vi "Down Hole CAL_PRESSURE_TRANSDUCER 2016.vi"(0 "Distance from APS Tip to transducer (ft)":dbl=5.2 format="%.2f", 2 "Sensor Cluster":T1, 3 "Descriptions":string[](array[string]), 5 "error in (no error)":errorcluster, 8 "Array in":refnum<k24>[](array[refnum])) -> (7 "DHT Zero (V)":dbl format="%.2f", 9 "DHT 10psi  (V)":dbl format="%.2f", 10 "Array out":refnum<k24>[](array[refnum]), 11 "DHT 50psi  (V)":dbl format="%.2f", 12 "Distance from APS Tip to transducer out":dbl=5.2 format="%.2f", 14 "Pressure\nSlope (psi/V)":dbl format="%.2f", 15 "Pressure\nOffset (psi)":dbl format="%.2f", 16 "Sensor Cluster 2":T1, 19 "error out":errorcluster)   [LabVIEW 2016]
uses:
  controls/MCC DAQ Readings.ctl
  C:/Cascade-lv16-64/builds/Waterloo Main Program/cascade/data/ULx_LV.dll
  builds/Waterloo Main Program/cascade/data/ULx_LV.dll
  Kpro Globals.vi
panel:
  in  "Exit":bool
  in  "50psi Pressure (psi)":dbl format="%.2f"
  in  "10psi Up Pressure (psi)":dbl format="%.2f"
  out "50psi indicator":bool
  in  "50psi button":bool
  out "Loop Counter":i32
  out "10psi\nindicator":bool
  out "zero indicator":bool
  in  "10psi button":bool
  in  "zero button":bool
  # "DOWNHOLE PRESSURE TRANSDUCER CALIBRATION"
  # "1. Connect the transducer to the KPRO line with the 3 way valve connected to the effluent of the transducer.  \n2.  Enter the distance from the APS tip to the transducer.\n3.  With the flow off, select the \"Record Zero Pressure\" button."
  # "3. Set the regulator pressure to a value close to 10psi, turn on the flow, close the 3-way valve and wait for the pressure to stabilize.  When it is stable, enter the \"10psi Pressure\" control, and select the \"Record ~10psi Voltage\" button."
  # "4. Set the regulator pressure to a value close to 50psi, turn on the flow, close the 3-way valve and wait for the pressure to stabilize.  When it is stable, enter the \"50psi Pressure\" control, and select the \"Record ~50psi Voltage\" button."
  # "5.  Slope and offset will be calculated, automatically.\nRecord the values for zero, slope and offset to the logbook and to the paper field log, then select the \"Record Values and Exit\" button."
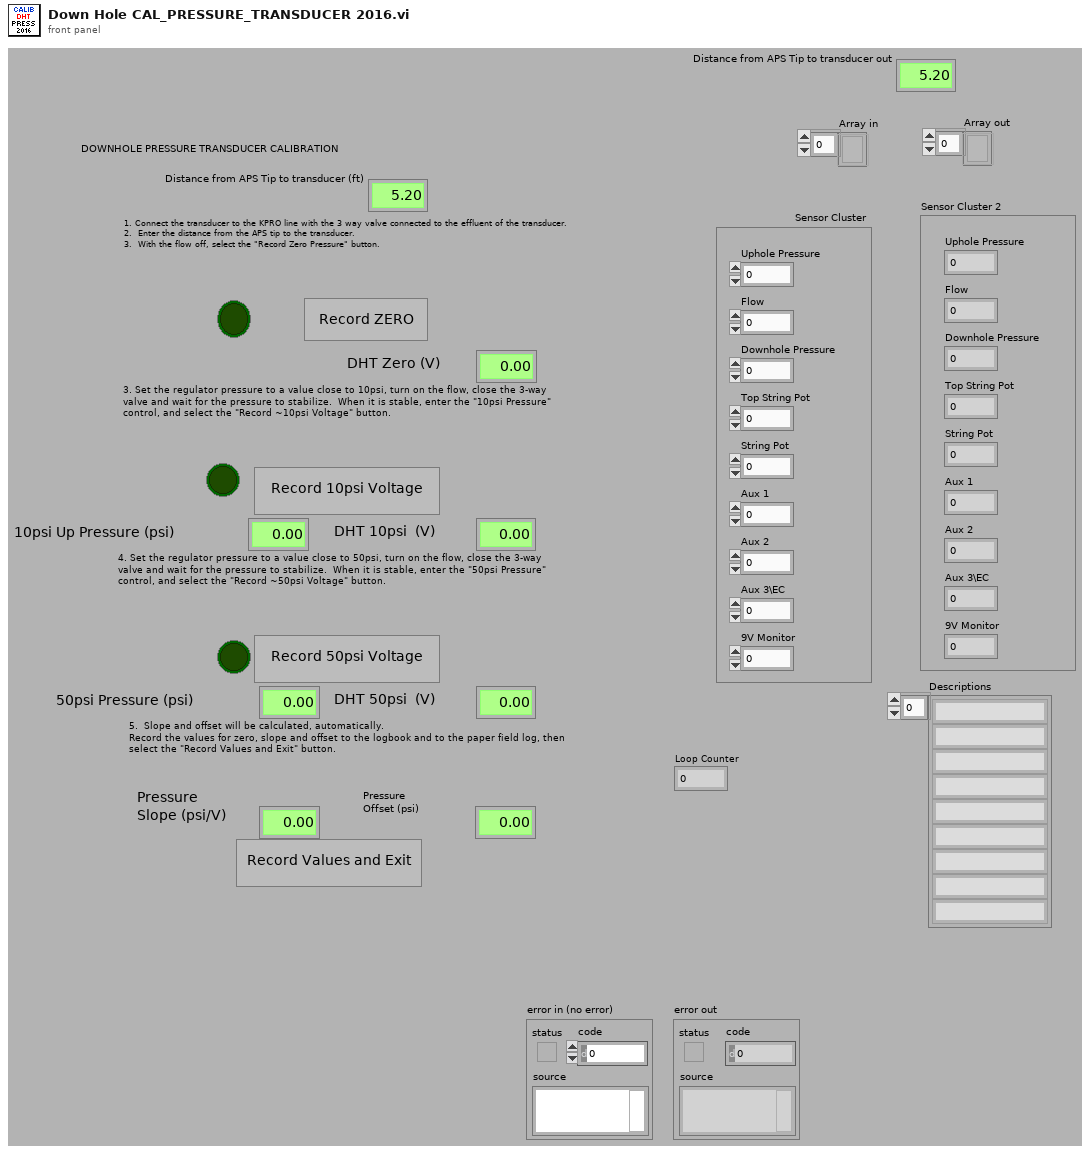
[diagram p1: front panel]
types:
  T1 = typedef "MCC DAQ Readings.ctl" = cluster{"Uphole Pressure":dbl, "Flow":dbl, "Downhole Pressure":dbl, "Top String Pot":dbl, "String Pot":dbl, "Aux 1":dbl, "Aux 2":dbl, "Aux 3\\EC":dbl, "9V Monitor":dbl}
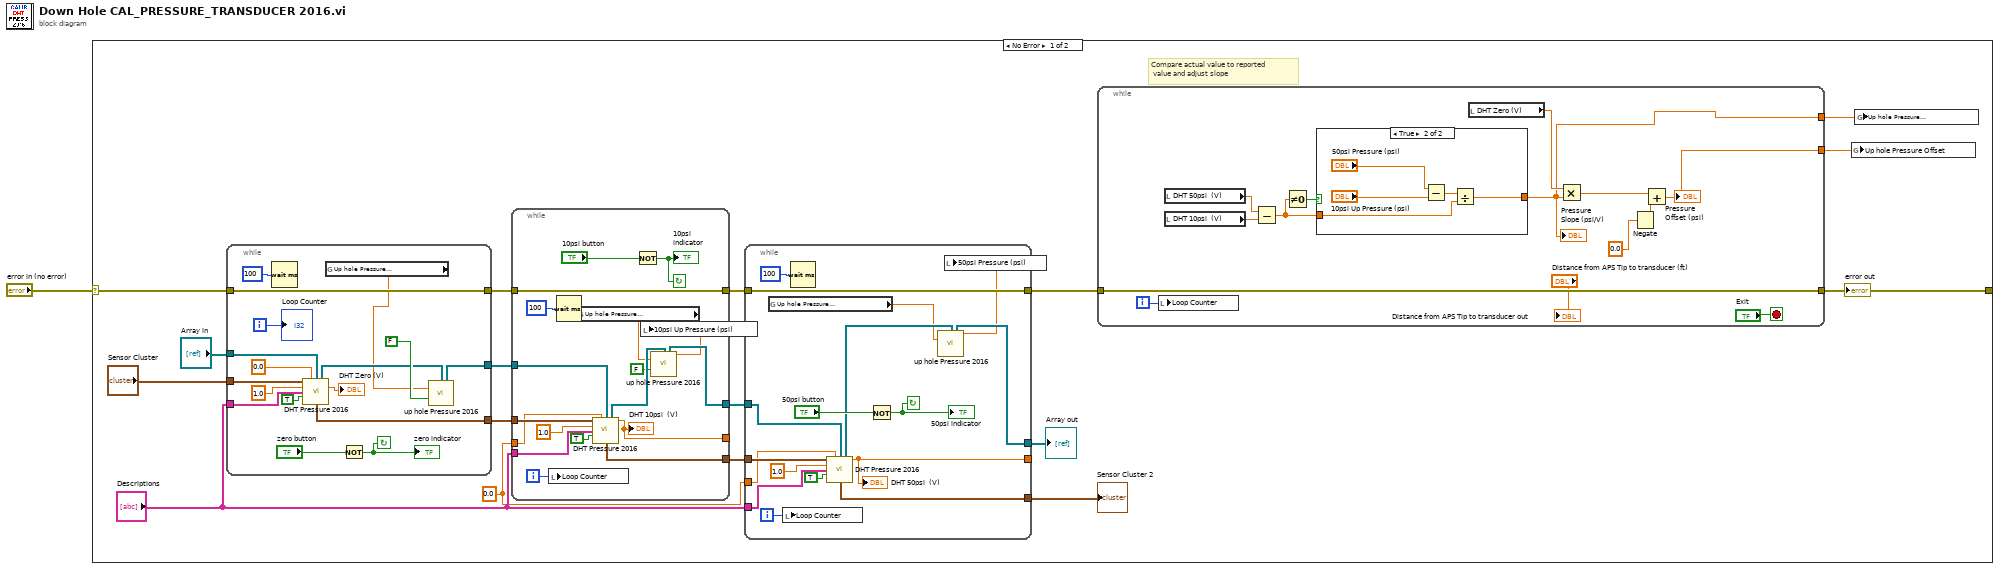
[diagram p0: block diagram]
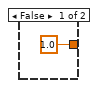
[diagram p2: hidden frame]
diagram:
  n1 = case shown="No Error" "error in (no error)" {
    selector: "error in (no error)" -> [w19 w92]
    tunnel: [w6 w92] -> w2
    frame No Error {
      w5 = 0.0
      # "Compare actual value to reported\n value and adjust slope"
      n2 = while {
        tunnel: [w72] -> w18
        tunnel: w19 -> [w72]
        tunnel: "Sensor Cluster" -> [w69]
        tunnel: "Array in" -> [w68]
        tunnel: [w58] -> w16
        tunnel: "Descriptions" -> [w67]
        tunnel: [w66] -> w14
        i -> [w62]
        stop <- w70 continue-if-true
        n3 = Wait (ms)(milliseconds to wait=u32 100) -> ()  [unwired: 1 out]
        n4 = call "DHT Pressure 2016.vi"("Sensor Cluster"=w69, "DHT Pressure Offset"=0.0, "Array in"=w68, "DHT Pressure \nSlope"=1.0 ("DHT Pressure \nSlope"), "Descriptions"=w67, "Zero Pressure\n(F = leave as is)"=TRUE ("Zero Pressure\n(F = leave as is)")) -> ("Array out"=w59:refnum<k24>[], "DHT Pressure (V)"=→"DHT Zero (V)":dbl, "Sensor Cluster 2"=w66:T1)  [unwired: 6 in, 1 out]
        n5 = global read "Kpro Globals.vi" "Up hole Pressure \nSlope"() -> (w57:dbl)
        n6 = Not(x="zero button") -> (.not. x?=w70:bool)
        "zero indicator" <- w70
        n7 = call "up hole Pressure 2016.vi"("Array in"=w59, "Pressure \nSlope"=w57, "Zero Pressure\n(F = leave as is)"=FALSE ("Zero Pressure\n(F = leave as is)")) -> ("Array out"=w58:refnum<k24>[])  [unwired: 9 in, 3 out]
        "Loop Counter" <- w62
      }
      n8 = while {
        tunnel: [w82] -> _
        tunnel: w18 -> [w90]
        tunnel: [w90] -> w13
        tunnel: w16 -> [w87]
        tunnel: [w77] -> w9
        tunnel: "Descriptions" -> [w86]
        tunnel: w14 -> [w85]
        tunnel: [w84] -> w12
        tunnel: w5 -> [w79]
        i -> [w80]
        stop <- w88 continue-if-true
        n9 = local write "Loop Counter"(w80) -> ()
        n10 = Wait (ms)(milliseconds to wait=u32 100) -> ()  [unwired: 1 out]
        n11 = global read "Kpro Globals.vi" "Up hole Pressure \nSlope"() -> (w76:dbl)
        n12 = call "DHT Pressure 2016.vi"("Sensor Cluster"=w85, "DHT Pressure Offset"=w79, "Array in"=w87, "DHT Pressure \nSlope"=1.0 ("DHT Pressure \nSlope"), "Descriptions"=w86, "Zero Pressure\n(F = leave as is)"=TRUE ("Zero Pressure\n(F = leave as is)")) -> ("Array out"=w78:refnum<k24>[], "DHT Pressure (ft/H20)"=w82:dbl, "Sensor Cluster 2"=w84:T1)  [unwired: 6 in, 1 out]
        "DHT 10psi  (V)" <- w82
        n13 = Not(x="10psi button") -> (.not. x?=w88:bool)
        "10psi\nindicator" <- w88
        n14 = call "up hole Pressure 2016.vi"("Array in"=w78, "Pressure \nSlope"=w76, "Zero Pressure\n(F = leave as is)"=FALSE ("Zero Pressure\n(F = leave as is)")) -> ("Array out"=w77:refnum<k24>[], "Uphole Pressure"=w74:dbl)  [unwired: 9 in, 2 out]
        n15 = local write "10psi Up Pressure (psi)"(w74) -> ()
      }
      n16 = while {
        tunnel: [w45] -> _
        tunnel: w13 -> [w56]
        tunnel: [w56] -> w7
        tunnel: w9 -> [w54]
        tunnel: [w43] -> w8
        tunnel: "Descriptions" -> [w53]
        tunnel: w12 -> [w52]
        tunnel: [w51] -> w10
        tunnel: w5 -> [w44]
        i -> [w46]
        stop <- w48 continue-if-true
        n17 = global read "Kpro Globals.vi" "Up hole Pressure \nSlope"() -> (w41:dbl)
        n18 = local write "Loop Counter"(w46) -> ()
        n19 = Wait (ms)(milliseconds to wait=u32 100) -> ()  [unwired: 1 out]
        n20 = call "DHT Pressure 2016.vi"("Sensor Cluster"=w52, "DHT Pressure Offset"=w44, "Array in"=w54, "DHT Pressure \nSlope"=1.0 ("DHT Pressure \nSlope"), "Descriptions"=w53, "Zero Pressure\n(F = leave as is)"=TRUE ("Zero Pressure\n(F = leave as is)")) -> ("Array out"=w42:refnum<k24>[], "DHT Pressure (ft/H20)"=w45:dbl, "Sensor Cluster 2"=w51:T1)  [unwired: 6 in, 1 out]
        "DHT 50psi  (V)" <- w45
        n21 = Not(x="50psi button") -> (.not. x?=w48:bool)
        "50psi indicator" <- w48
        n22 = call "up hole Pressure 2016.vi"("Array in"=w42, "Pressure \nSlope"=w41) -> ("Array out"=w43:refnum<k24>[], "Uphole Pressure"=w40:dbl)  [unwired: 10 in, 2 out]
        n23 = local write "50psi Pressure (psi)"(w40) -> ()
      }
      "Array out" <- w8
      "Sensor Cluster 2" <- w10
      n24 = while {
        tunnel: w7 -> [w31]
        tunnel: [w31] -> w6
        tunnel: [w21] -> w4
        tunnel: [w20] -> w3
        i -> [w24]
        stop <- "Exit" stop-if-true
        n25 = local write "Loop Counter"(w24) -> ()
        n26 = local read "DHT 50psi  (V)"() -> (w29:dbl)
        n27 = local read "DHT 10psi  (V)"() -> (w28:dbl)
        n28 = Subtract(x=w29, y=w28) -> (x-y=w33:dbl)
        n29 = Not Equal To 0?(x=w33) -> (x != 0?=w32:bool)
        n30 = case shown="True" w32 {
          tunnel: [1.0 w35] -> w21
          tunnel: w33 -> [_ w39]
          frame False {
          }
          frame True {
            n31 = Subtract(x="50psi Pressure (psi)", y="10psi Up Pressure (psi)") -> (x-y=w37:dbl)
            n32 = Divide(x=w37, y=w39) -> (x/y=w35:dbl)
          }
        }
        "Pressure\nSlope (psi/V)" <- w21
        n33 = local read "DHT Zero (V)"() -> (w27:dbl)
        n34 = Multiply(x=w27, y=w21) -> (x*y=w26:dbl)
        n35 = Negate(x=0.0) -> (-x=w23:dbl)
        n36 = Add(x=w26, y=w23) -> (x+y=w20:dbl)
        "Pressure\nOffset (psi)" <- w20
        "Distance from APS Tip to transducer out" <- "Distance from APS Tip to transducer (ft)"
      }
      n37 = global write "Kpro Globals.vi" "Up hole Pressure Offset"(w3) -> ()
      n38 = global write "Kpro Globals.vi" "Up hole Pressure \nSlope"(w4) -> ()
    }
    frame Error {
    }
  }
  "error out" <- w2
